vi "test_no_connector_pane.vi"() -> ()   [LabVIEW 2026]
panel:
  out "Sum":dbl
  in  "Input 2":dbl
  in  "Input 1":dbl
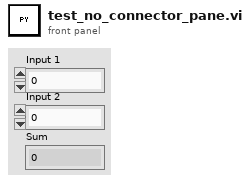
[diagram p1: front panel]
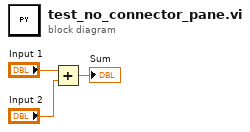
[diagram p0: block diagram]
diagram:
  n1 = Add(x="Input 1", y="Input 2") -> (x+y=→"Sum":dbl)
